vi "Generate Text Report.vi"(8 "error in (no error)":errorcluster, 10 "Storage":refnum<class "Test Event Storage.lvclass">, 11 "Basic Test Manager in":refnum<class "Basic Test Manager.lvclass">) -> (0 "error out":errorcluster, 2 "Report":string, 3 "Basic Test Manager out":refnum<class "Basic Test Manager.lvclass">)   [LabVIEW 2009, in "Caraya.lvlib" / "Basic Test Manager.lvclass"]
uses:
  Basic Test Manager.lvclass
  Test Event Storage/Test Event Storage.lvclass
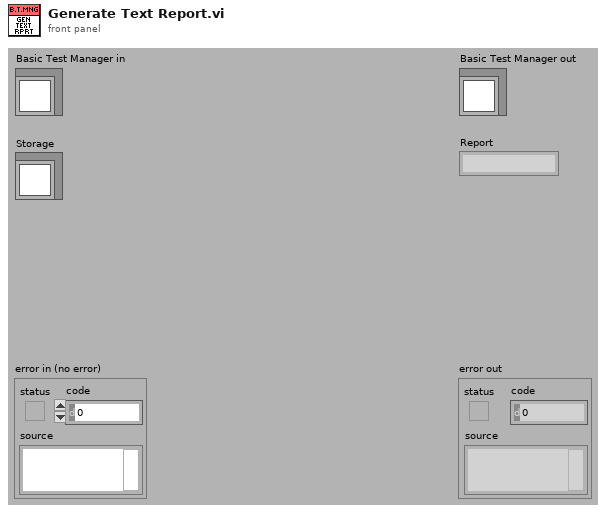
[diagram p1: front panel]
types:
  T1 = typedef "Caraya.lvlib/Test Event Storage.lvclass/Test Node.ctl" = cluster{"Test Registration":T2, "Defined":bool, "Passed":bool}
  T2 = typedef "Caraya.lvlib/Basic Test Manager.lvclass/Test Registration Data.ctl" = cluster{"Name":string, "Call Chain":string[], "Time Stamp":timestamp}
  T3 = typedef "Caraya.lvlib/Basic Test Manager.lvclass/Assert Event Data.ctl" = cluster{"Name":string, "Passed":bool, "Call Chain":string[], "Test Error":errorcluster, "Time Stamp":timestamp}
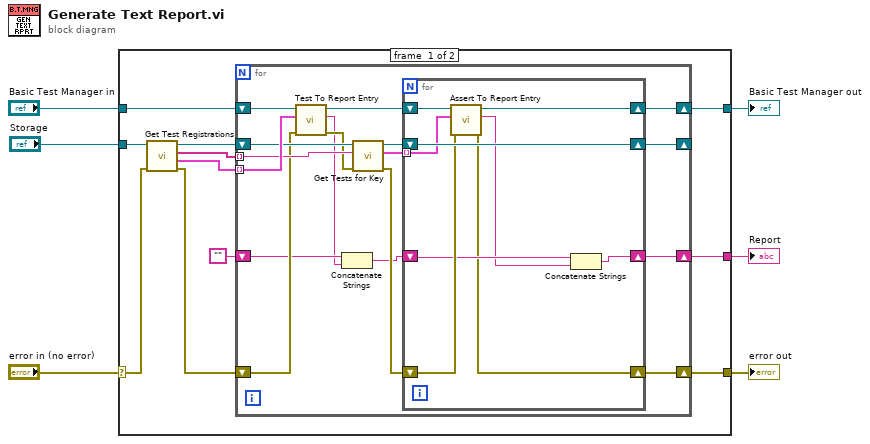
[diagram p0: block diagram]
diagram:
  n1 = case shown="No Error" "error in (no error)" {
    selector: "error in (no error)" -> [w11 w45]
    tunnel: [w9 w45] -> w5
    tunnel: [w8 w44] -> w3
    tunnel: "Basic Test Manager in" -> [w12 w44]
    tunnel: "Storage" -> [w17 _]
    tunnel: [w7 _] -> w1
    frame #0 {
      n2 = call-dynamic "Get Test Registrations.vi"("error in (no error)"=w11, "Test Event Storage in"=w17) -> ("error out"=w10:errorcluster, "Test Registrations"=w16:T1[], "Keys"=w15:string[], "Test Event Storage out"=w13:refnum<class "Test Event Storage.lvclass">)  [unwired: 5 in, 1 out]
      n3 = for {
        tunnel: w16 -> [w33] mode=indexing
        tunnel: w15 -> [w31] mode=indexing
        shift-right: [w23] -> w7
        shift-left: "" -> [w22]
        shift-right: [w18] -> _
        shift-left: w13 -> [w32]
        shift-right: [w24] -> w8
        shift-left: w12 -> [w34]
        shift-right: [w19] -> w9
        shift-left: w10 -> [w30]
        n4 = call "Test To Report Entry.vi"("error in (no error)"=w30, "Test Node"=w33, "Basic Test Manager in"=w34) -> ("error out"=w29:errorcluster, "String"=w20:string, "Basic Test Manager out"=w28:refnum<class "Basic Test Manager.lvclass">)  [unwired: 6 in]
        n5 = Concatenate Strings(w22, w20) -> (w21:string)
        n6 = call "Get Tests for Key.vi"("error in (no error)"=w29, "Key"=w31, "Test Event Storage in"=w32) -> ("error out"=w26:errorcluster, "Test Events"=w25:T3[], "Test Event Storage out"=w27:refnum<class "Test Event Storage.lvclass">)  [unwired: 6 in]
        n7 = for {
          shift-right: [w38] -> w24
          shift-left: w28 -> [w42]
          shift-right: [w43] -> w18
          shift-left: w27 -> [w43]
          shift-right: [w35] -> w19
          shift-left: w26 -> [w40]
          tunnel: w25 -> [w41] mode=indexing
          shift-right: [w36] -> w23
          shift-left: w21 -> [w39]
          n8 = call "Assert To Report Entry.vi"("error in (no error)"=w40, "Assert"=w41, "Basic Test Manager in"=w42) -> ("error out"=w35:errorcluster, "String"=w37:string, "Basic Test Manager out"=w38:refnum<class "Basic Test Manager.lvclass">)  [unwired: 6 in]
          n9 = Concatenate Strings(w39, w37) -> (w36:string)
        }
      }
    }
    frame #1 {
    }
  }
  "error out" <- w5
  "Basic Test Manager out" <- w3
  "Report" <- w1
